vi "MCConfigBrakeSingle.vi"(8 "error in (no error)":errorcluster, 10 "MotorConfig":T1={"CAN Address"=0, "Invert"=FALSE, "InvertSensor"=FALSE, "Unit Conversion Factor"=0.0, "Brake Mode"=enum."Override to Brake", "Reverse Limt Switch Mode"=enum."Disabled", "Forward Limt Swith Mode"=enum."Disabled", "PWM Channel"=enum."Invalid", "Motor Controller Type"=enum."Talon SRX", "Peak Current (A)"=0, "Continuous Current (A)"=0, "Peak Duration (ms)"=0, "Current Limit Enable"=FALSE}, 11 "PhoenixMotorControlDevRefIn":T6={"DeviceStatus"={"status"=FALSE, "code"=0, "source"=""}, "Type"=enum."PWM", "PWM"={"PWM Channel"=enum."PWM 1", "DeadBand"={"Name"="", "maxPositivePwm"=0, "minPositivePwm"=0, "centerPwm"=0, "maxNegativePwm"=0, "minNegativePwm"=0, "angularRange"=0}}, "CAN"={"Device Number"=0, "SetOutput VI Ref"=variant(enum8{"Percent VBus", "Current", "Speed", "Position", "Voltage"} enum."Percent VBus"), "GetOutput VI Ref"=variant(refnum<k1> refnum), "Enable VI Ref"=variant(dbl 12.0), "Disable VI Ref"=variant(enum8{"Percent VBus", "Speed", "Position", "Slave", "Unchanged / Invalid", "Voltage Compensation", "Current", "Motion Profile"} enum."Percent VBus"), "Data"=variant}, "Invert"=FALSE, "DIO PWM"={"PWM \"Enable\" Channel"=enum."Invalid", "DIOChannel"=enum."Invalid", "PWM Rate"=0.0}}) -> (0 "error out":errorcluster, 3 "PhoenixMotorControlDevRefOut":T6={"DeviceStatus"={"status"=FALSE, "code"=0, "source"=""}, "Type"=enum."PWM", "PWM"={"PWM Channel"=enum."PWM 1", "DeadBand"={"Name"="", "maxPositivePwm"=0, "minPositivePwm"=0, "centerPwm"=0, "maxNegativePwm"=0, "minNegativePwm"=0, "angularRange"=0}}, "CAN"={"Device Number"=0, "SetOutput VI Ref"=variant(enum8{"Percent VBus", "Current", "Speed", "Position", "Voltage"} enum."Percent VBus"), "GetOutput VI Ref"=variant(refnum<k1> refnum), "Enable VI Ref"=variant(dbl 12.0), "Disable VI Ref"=variant(enum8{"Percent VBus", "Speed", "Position", "Slave", "Unchanged / Invalid", "Voltage Compensation", "Current", "Motion Profile"} enum."Percent VBus"), "Data"=variant}, "Invert"=FALSE, "DIO PWM"={"PWM \"Enable\" Channel"=enum."Invalid", "DIOChannel"=enum."Invalid", "PWM Rate"=0.0}})   [LabVIEW 2019, in "ArgosLib.lvlib"]
uses:
  ArgosLib.lvlib
  <vilib>/Rock Robotics/WPI/MotorControl/WPI_MotorControlDeviceRef.ctl
  <vilib>/Rock Robotics/WPI/MotorControl/WPI_MotorControlType.ctl
  <vilib>/Rock Robotics/SystemInterfaces/DIO/FPGA_DIOPWMChannel.ctl
  <vilib>/Rock Robotics/WPI/PWM/WPI_PWMDeadband.ctl
  <vilib>/Rock Robotics/SystemInterfaces/DIO/FPGA_DIOChannel.ctl
  Config/ConfigComponents/TypeDefs/Config_Motor.ctl
  <vilib>/Rock Robotics/WPI/ThirdParty/Phoenix-LabVIEW/Motor Controller/Controls/CTRE_Phoenix_MotorControl_NeutralMode.ctl
  <vilib>/Rock Robotics/WPI/ThirdParty/Phoenix-LabVIEW/Motor Controller/Controls/CTRE_Phoenix_MotorControl_LimitSwitchNormal.ctl
  Config/ConfigComponents/TypeDefs/Config_MotorCtrlType.ctl
  <vilib>/Playing With Fusion Inc/Playing With Fusion Lib for FRC/PWF_Venom_LabVIEW/Public/TypeDefs/PwF_Venom_BrakeCoastMode.ctl
  <vilib>/Playing With Fusion Inc/Playing With Fusion Lib for FRC/PWF_Venom_LabVIEW/PwF_Venom.lvlib
  <vilib>/Rock Robotics/WPI/ThirdParty/REV Robotics/SPARK MAX/Typedef/Spark MAX Idle Mode.ctl
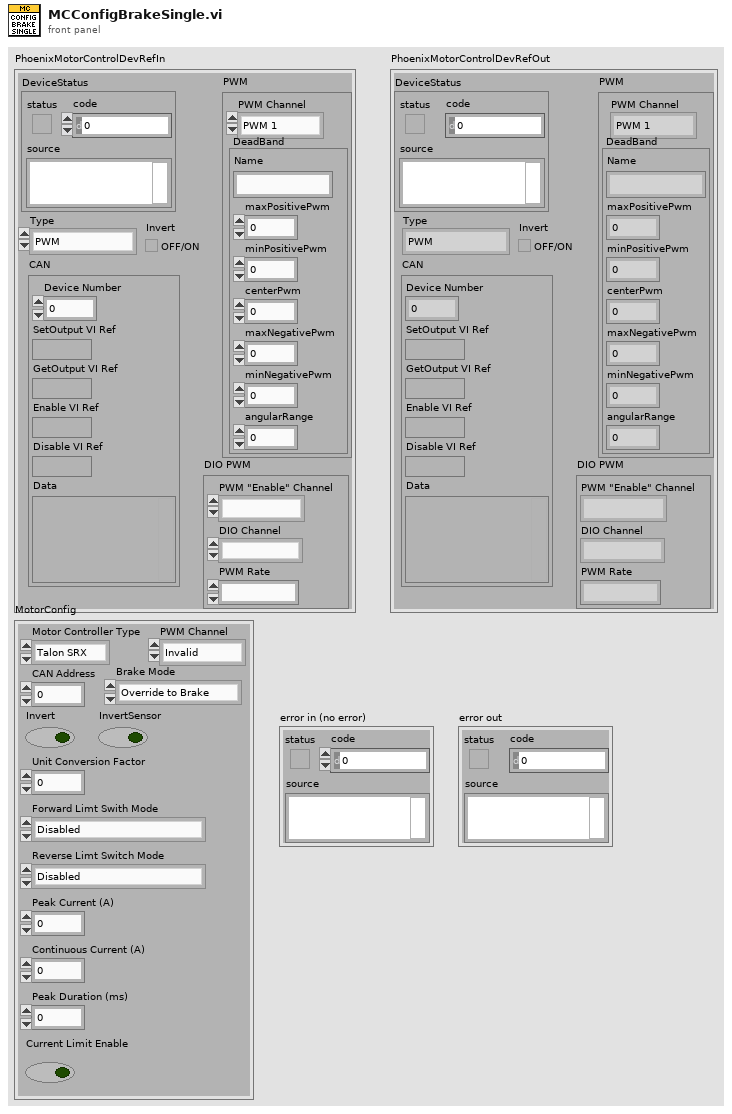
[diagram p1: front panel]
types:
  T1 = typedef "ArgosLib.lvlib/Config_Motor.ctl" = cluster{"CAN Address":u8, "Invert":bool, "InvertSensor":bool, "Unit Conversion Factor":dbl, "Brake Mode":T2, "Reverse Limt Switch Mode":T3, "Forward Limt Swith Mode":T3, "PWM Channel":T4, "Motor Controller Type":T5, "Peak Current (A)":i32, "Continuous Current (A)":i32, "Peak Duration (ms)":i32, "Current Limit Enable":bool}
  T2 = typedef "CTRE_Phoenix_MotorControl_NeutralMode.ctl" = enum8{"EEPROMSetting", "Override to Coast", "Override to Brake"}
  T3 = typedef "CTRE_Phoenix_MotorControl_LimitSwitchNormal.ctl" = enum16{"Normally Open", "Normally Closed", "Disabled"}
  T4 = typedef "FPGA_DIOPWMChannel.ctl" = enum8{"PWM 0", "PWM 1", "PWM 2", "PWM 3", "PWM 4", "PWM 5", "PWM 6", "PWM 7", "PWM 8", "PWM 9", "PWM MXP 0", "PWM MXP 1", "PWM MXP 2", "PWM MXP 3", "PWM MXP 4", "PWM MXP 5", "PWM MXP 6", "PWM MXP 7", "PWM MXP 8", "PWM MXP 9", "Invalid"}
  T5 = typedef "ArgosLib.lvlib/Config_MotorCtrlType.ctl" = enum16{"Disabled", "Talon SRX", "Talon SR", "Venom", "Spark MAX"}
  T6 = typedef "WPI_MotorControlDeviceRef.ctl" = cluster{"DeviceStatus":errorcluster, "Type":T7, "PWM":cluster{"PWM Channel":T4, "DeadBand":T8}, "CAN":cluster{"Device Number":u8, "SetOutput VI Ref":variant, "GetOutput VI Ref":variant, "Enable VI Ref":variant, "Disable VI Ref":variant, "Data":variant}, "Invert":bool, "DIO PWM":cluster{"PWM \"Enable\" Channel":T4, "DIOChannel":T9, "PWM Rate":dbl}}
  T7 = typedef "WPI_MotorControlType.ctl" = enum16{"PWM", "CAN", "DIO PWM"}
  T8 = typedef "WPI_PWMDeadband.ctl" = cluster{"Name":string, "maxPositivePwm":i32, "minPositivePwm":i32, "centerPwm":i32, "maxNegativePwm":i32, "minNegativePwm":i32, "angularRange":u16}
  T9 = typedef "FPGA_DIOChannel.ctl" = enum8{"DIO 0", "DIO 1", "DIO 2", "DIO 3", "DIO 4", "DIO 5", "DIO 6", "DIO 7", "DIO 8", "DIO 9", "DIO MXP 0", "DIO MXP 1", "DIO MXP 2", "DIO MXP 3", "DIO MXP 4", "DIO MXP 5", "DIO MXP 6", "DIO MXP 7", "DIO MXP 8", "DIO MXP 9", "DIO MXP 10", "DIO MXP 11", "DIO MXP 12", "DIO MXP 13", "DIO MXP 14", "DIO MXP 15", "SPI Port CS1", "SPI Port CS2", "SPI Port CS3", "SPI Port MISO", "SPI Port MOSI", "Invalid"}
  T10 = typedef "Spark MAX Idle Mode.ctl" = enum16{"Coast", "Brake"}
  T11 = typedef "PlayingWithFusionLib.lvlib/PwF_Venom.lvlib/PwF_Venom_BrakeCoastMode.ctl" = u8
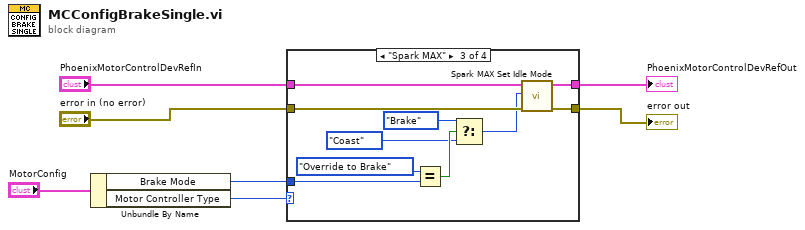
[diagram p0: block diagram]
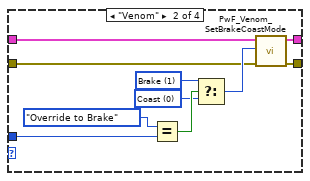
[diagram p3: hidden frame]
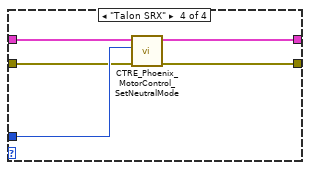
[diagram p4: hidden frame]
diagram:
  n1 = Unbundle By Name("MotorConfig") -> ("Brake Mode"=w6:T2, "Motor Controller Type"=w1:T5)
  n2 = case shown="\"Spark MAX\"" w1 {
    tunnel: w6 -> [_ w16 w25 w34]
    tunnel: "PhoenixMotorControlDevRefIn" -> [w9 w19 w29 w33]
    tunnel: [w9 w18 w28 w32] -> w4
    tunnel: "error in (no error)" -> [w8 w10 w27 w31]
    tunnel: [w8 w17 w26 w30] -> w2
    frame "Disabled", Default {
    }
    frame "Venom" {
      w12 = T11 1 items=["Coast", "Brake"] ("t")
      w13 = T11 0 items=["Coast", "Brake"] ("Brake Coast Mode")
      n3 = Equal?(x=CTRE_Phoenix_MotorControl_NeutralMode."Override to Brake", y=w16) -> (x = y?=w14:bool)
      n4 = Select(t=w12, s=w14, f=w13) -> (s? t:f=w11:T11)
      n5 = call <vilib>:"PwF_Venom_SetBrakeCoastMode.vi"("error in"=w10, "Brake Coast Mode"=w11, "PwFVenomDevRefIn"=w19) -> ("error out"=w17:errorcluster, "PwFVenomDevRefOut"=w18:T6)  [unwired: 7 in]
    }
    frame "Spark MAX" {
      n6 = Equal?(x=CTRE_Phoenix_MotorControl_NeutralMode."Override to Brake", y=w25) -> (x = y?=w23:bool)
      n7 = Select(t=Spark_MAX_Idle_Mode."Brake", s=w23, f=Spark_MAX_Idle_Mode."Coast" ("Idle Mode")) -> (s? t:f=w20:T10)
      n8 = call <vilib>:"Spark MAX Set Idle Mode.vi"("error in (no error)"=w27, "Idle Mode"=w20, "MotorControlDeviceRef in"=w29) -> ("error out"=w26:errorcluster, "MotorControlDeviceRef out"=w28:T6)  [unwired: 7 in]
    }
    frame "Talon SRX" {
      n9 = call <vilib>:"CTRE_Phoenix_MotorControl_SetNeutralMode.vi"("error in (no error)"=w31, "Motor Control Neutral Mode"=w34, "PhoenixMotorControlDevRef"=w33) -> ("error out"=w30:errorcluster, "PhoenixMotorControlDevRef"=w32:T6)  [unwired: 7 in]
    }
  }
  "PhoenixMotorControlDevRefOut" <- w4
  "error out" <- w2
